vi "SshKeywordReadBinary.vi"(0 "error in (no error)":errorcluster, 5 "Pattern":string, 6 "SshStream in":refnum<k24>, 7 "Service":string, 9 "Keyword":string) -> (2 "Result":string, 3 "error out":errorcluster, 10 "SshStream out":refnum<k24>)   [LabVIEW 2009]
uses:
  C:/Ohana/LV2009/OhanaOS-LV81/Instruments/Keyword/Controller/Tamir.sharpSsh.dll
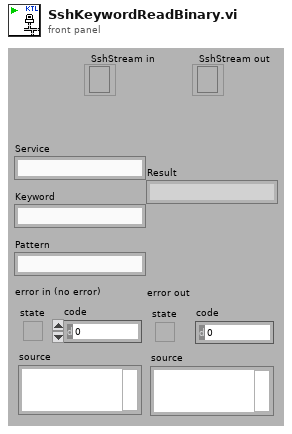
[diagram p1: front panel]
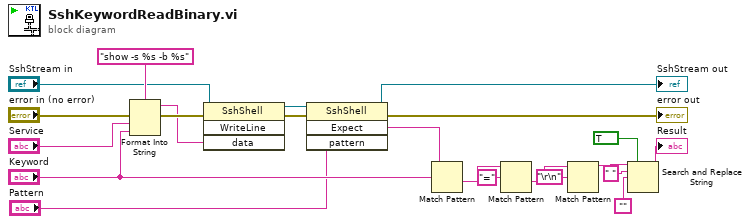
[diagram p0: block diagram]
diagram:
  n1 = Format Into String(format string="show -s %s -b %s" ("data"), error in="error in (no error)", "Service", "Keyword") -> (resulting string=w4:string, error out=w21:errorcluster)  [unwired: 1 in]
  n2 = invoke class="SshShell" method="WriteLine"(reference="SshStream in", error in=w21, "data"=w4) -> (reference out=w3:refnum<k24>, error out=w18:errorcluster)  [unwired: 1 in, 2 out]
  n3 = invoke class="SshShell" method="Expect"(reference=w3, error in=w18, "pattern"="Pattern") -> (reference out=→"SshStream out":refnum<k24>, error out=→"error out":errorcluster, "Expect"=w2:string)  [unwired: 1 in, 1 out]
  n4 = Match Pattern(string=w2, regular expression="Keyword") -> (after substring=w13:string)  [unwired: 4 out]
  n5 = Match Pattern(string=w13, regular expression="=" ("expression régulière")) -> (after substring=w11:string)  [unwired: 4 out]
  n6 = Match Pattern(string=w11, regular expression="\r\n" ("expression régulière")) -> (before substring=w10:string)  [unwired: 4 out]
  n7 = Search and Replace String(replace all?=TRUE ("tout remplacer ? (F)"), input string=w10, search string=" " ("chaîne recherchée"), replace string="") -> (result string=→"Result":string)  [unwired: 1 in, 6 out]
